vi "create GUID.vi"() -> (3 "uuid":string)   [LabVIEW 2013, in "NISE_CEF_serializable configuration.lvclass"]
doc: "Generates a unique identification string"
uses:
  NISE_CEF_serializable configuration.lvclass
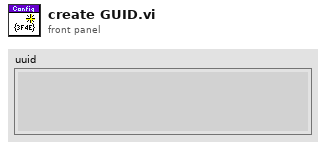
[diagram p1: front panel]
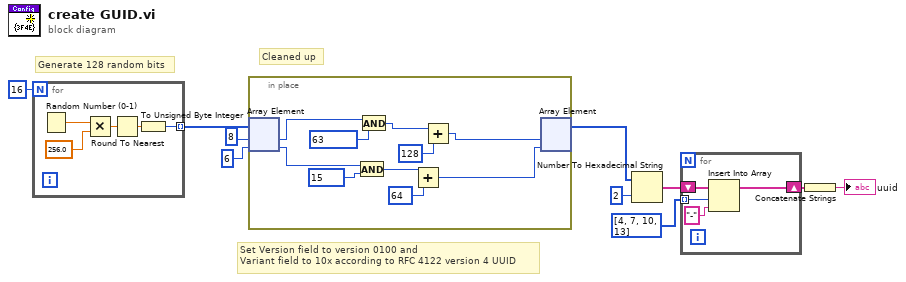
[diagram p0: block diagram]
diagram:
  # "Cleaned up"
  # "Set Version field to version 0100 and \nVariant field to 10x according to RFC 4122 version 4 UUID"
  # "Generate 128 random bits"
  n1 = for {
    N: 16 -> [_]
    tunnel: [w11] -> w8 mode=indexing
    n2 = Random Number (0-1)() -> (number: 0 to 1=w15:dbl)
    n3 = Multiply(x=w15, y=256.0) -> (x*y=w13:dbl)
    n4 = Round To Nearest(number=w13) -> (nearest integer value=w12:dbl)
    n5 = To Unsigned Byte Integer(number=w12) -> (unsigned 8bit integer=w11:u8)
  }
  n6 = in-place {
    n7 = in-place-array #1(w8, 8 ("index"), 6 ("index")) -> (w24:u8, w23:u8)
    n8 = And(x=w23, y=u8 15) -> (x .and. y?=w20:u8)
    n9 = And(x=w24, y=u8 63) -> (x .and. y?=w18:u8)
    n10 = Add(x=w20, y=u8 64) -> (x+y=w16:u8)
    n11 = Add(x=w18, y=u8 128) -> (x+y=w17:u8)
    n12 = in-place-array #1(w17, w16) -> (w10:u8[])  [unwired: 2 out]
  }
  n13 = Number To Hexadecimal String(1:i16 2 ("width (-)"), 2:w10) -> (0:w6:string[])
  n14 = for {
    shift-right: [w28] -> w5
    shift-left: w6 -> [w29]
    tunnel: i32[] [4, 7, 10, 13] ("Array") -> [w26] mode=indexing
    n15 = Insert Into Array(array=w29, index=w26, new element="-" ("new element/subarray")) -> (w28:string[])
  }
  n16 = Concatenate Strings(w5) -> (→"uuid":string)
